vi "Find_FPGA_Build_Specs.vi"(11 "Application in":refnum<vi>) -> (3 "Build Spec Details":T1(array[cluster]))   [LabVIEW 2013]
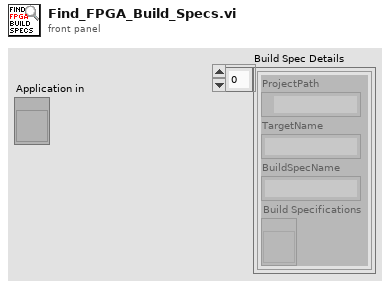
[diagram p1: front panel]
types:
  T1 = cluster{"ProjectPath":path, "TargetName":string, "BuildSpecName":string, "Build Specifications":refnum<vi>}[]
  T2 = cluster{"ProjectPath":path, "TargetName":string, "BuildSpecName":string, "Build Specifications":refnum<vi>}
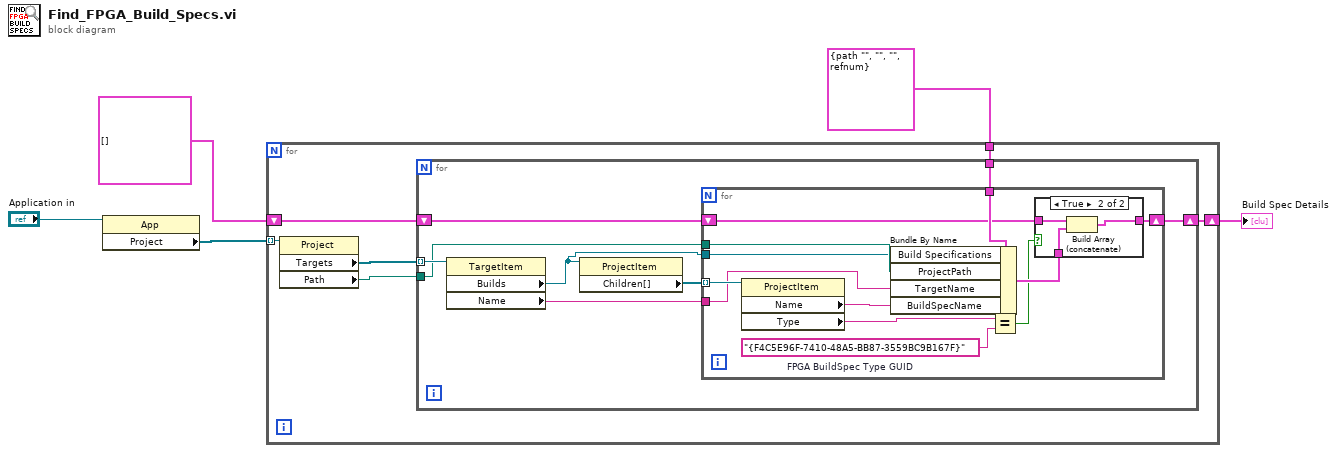
[diagram p0: block diagram]
diagram:
  n1 = property class="App"(reference="Application in") -> ("Project"=w4:refnum<vi>[])  [unwired: 1 in, 2 out]
  n2 = for {
    tunnel: w4 -> [w8] mode=indexing
    shift-right: [w10] -> w3
    shift-left: T1 [] -> [w7]
    tunnel: T2 {"ProjectPath"=path "", "TargetName"="", "BuildSpecName"="", "Build Specifications"=refnum} ("build spec path") -> [w6]
    n3 = property class="Project"(reference=w8) -> ("Targets"=w11:refnum<vi>[], "Path"=w9:path)  [unwired: 1 in, 2 out]
    n4 = for {
      tunnel: w11 -> [w19] mode=indexing
      shift-right: [w13] -> w10
      shift-left: w7 -> [w14]
      tunnel: w9 -> [w16]
      tunnel: w6 -> [w15]
      n5 = property class="TargetItem"(reference=w19) -> ("Builds"=w12:refnum<vi>, "Name"=w17:string)  [unwired: 1 in, 2 out]
      n6 = property class="ProjectItem"(reference=w12) -> ("Children[]"=w18:refnum<vi>[])  [unwired: 1 in, 2 out]
      n7 = for {
        tunnel: w18 -> [w31] mode=indexing
        tunnel: w17 -> [w28]
        tunnel: w16 -> [w30]
        tunnel: w15 -> [w27]
        shift-right: [w25] -> w13
        shift-left: w14 -> [w26]
        tunnel: w12 -> [w20]
        w23 = "{F4C5E96F-7410-48A5-BB87-3559BC9B167F}"  # FPGA BuildSpec Type GUID
        n8 = property class="ProjectItem"(reference=w31) -> ("Name"=w29:string, "Type"=w22:string)  [unwired: 1 in, 2 out]
        n9 = Bundle By Name(cluster=w27, "Build Specifications"=w20, "ProjectPath"=w30, "TargetName"=w28, "BuildSpecName"=w29) -> (w24:T2)
        n10 = Equal?(x=w22, y=w23) -> (x = y?=w21:bool)
        n11 = case shown="True" w21 {
          tunnel: w26 -> [w32 w35]
          tunnel: [w32 w33] -> w25
          tunnel: w24 -> [_ w34]
          frame False {
          }
          frame True {
            n12 = Build Array (concatenate)(w35, w34) -> (w33:T1)
          }
        }
      }
    }
  }
  "Build Spec Details" <- w3
